vi "TestHyperdata.vi"() -> ()   [LabVIEW 2009]
panel:
  in  "dimension size":i32=600
  out "Test Run No CLR":dbl[](array[numeric])=[4.796875, 6.515625, 1.796875, 0.484375, 3.0, 3.0, 6.21875, 1.1875, 8.234375, 7.625, 2.984375, 2.5, 1.890625, 8.625, 4.296875, 0.578125, 3.890625, 1.78125, 2.0, 3.0]
  out "Array 4":dbl[](array[numeric])
  out "Array 3":i32[](array[numeric])
  out "Elapsed Time (sec)":dbl format="%.2f"
  out "Array 2":errorcluster[](array[cluster])
  out "Array":dbl[](array[numeric])
  out "Error Out":errorcluster
  in  "ComPort":refnum<visa-resource-name>="COM1"
  out "GEA2 Hyperdata":string
  out "Numeric":i32
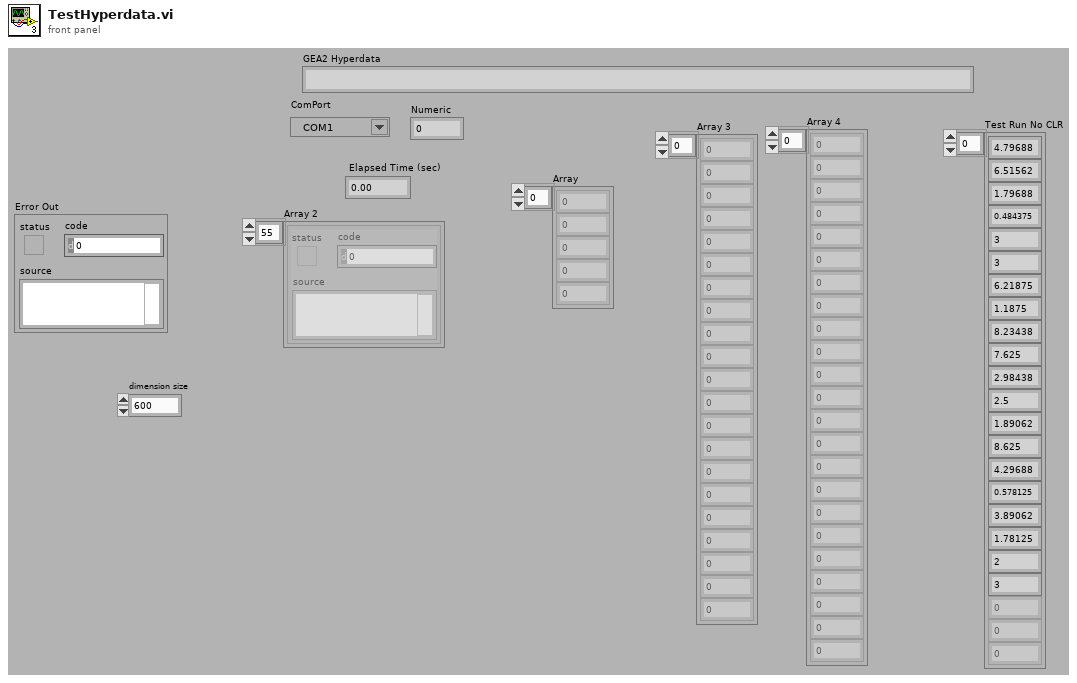
[diagram p1: front panel]
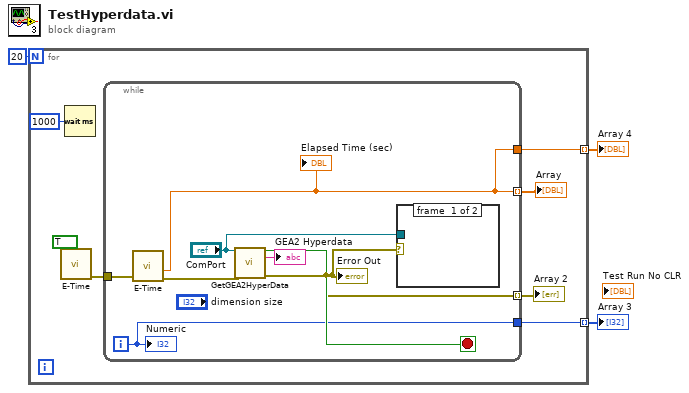
[diagram p0: block diagram]
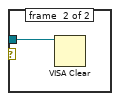
[diagram p2: hidden frame]
diagram:
  n1 = for {
    N: 20 -> [_]
    tunnel: [w8] -> w2 mode=indexing
    tunnel: [w5] -> w1 mode=indexing
    n2 = call "E-Time.vi"("Reset"=TRUE) -> ("error out"=w7:errorcluster)  [unwired: 8 in, 2 out]
    n3 = Wait (ms)(milliseconds to wait=u32 1000) -> ()  [unwired: 1 out]
    n4 = while {
      tunnel: [w12] -> w9 mode=indexing
      tunnel: [w13] -> w10 mode=indexing
      tunnel: [w15] -> w8
      tunnel: w7 -> [w14]
      tunnel: [w13] -> w5
      i -> [w15]
      stop <- w18 stop-if-true
      n5 = call "E-Time.vi"("error in (no error)"=w14) -> ("error out"=w16:errorcluster, "Elapsed Time (sec)"=w13:dbl)  [unwired: 8 in, 1 out]
      "Elapsed Time (sec)" <- w13
      n6 = call "GetGEA2HyperData.vi"("ComPort"="ComPort", "Error In"=w16) -> ("ACK"=w18:bool, "GEA2 Hyperdata"=→"GEA2 Hyperdata":string, "Error Out"=w12:errorcluster)  [unwired: 11 in]
      "Error Out" <- w12
      n7 = case shown="Error" w12 {
        tunnel: "ComPort" -> [_ w19]
        frame #0 {
        }
        frame #1 {
          n8 = VISA Clear(VISA resource name=w19) -> ()  [unwired: 1 in, 2 out]
        }
      }
      "Numeric" <- w15
    }
    "Array" <- w10
    "Array 2" <- w9
  }
  "Array 3" <- w2
  "Array 4" <- w1
